vi "_Yt10_GoTo.vi"(11 "YTESTER测试数据":T1) -> (3 "YTESTER结论":T2)   [LabVIEW 2017]
doc: "VIClassID=YT_SSTEPFLAG_GOTO\nVIDescription=如果前面失败的话可以跳转某一位置进行重测，测试表也会更新掉。注意，也可以往后跳"
uses:
  YtCommon.lvlibp/yt`Step StepBaseInput.ctl
  YtCommon.lvlibp/yt`Step StepResult.ctl
  YtCommon.lvlibp/yt`Step TestData.ctl
  YtCommon.lvlibp/yt`Step System Queue.ctl
  YtCommon.lvlibp
panel:
  in  "YTESTER开放参数":T4={"YTESTER_BaseInput"={"isTest"=FALSE, "isSkip"=FALSE, "StepName"="Goto跳转器", "OnPass"=enum."Next", "OnFail"=enum."Next", "ReTestNumber"=0.0}, "跳转目标行(from1)"=1}
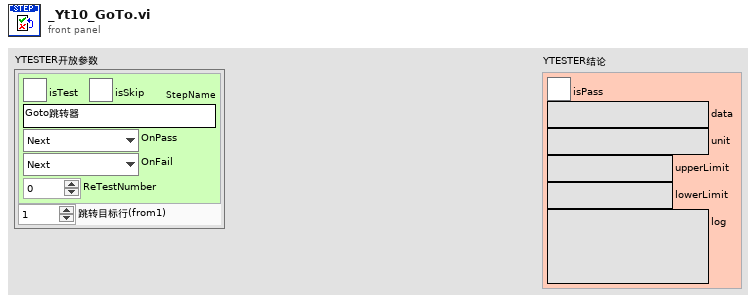
[diagram p1: front panel]
types:
  T1 = typedef "YtCommon.lvlibp/yt`Step TestData.ctl" = cluster{"Socket(From1)":i32, "SN":refnum<notifier>, "StopFlagRef":refnum<notifier>, "YT System Queue":refnum<queue>}
  T2 = typedef "YtCommon.lvlibp/yt`Step StepResult.ctl" = cluster{"isPass":bool, "data":string, "unit":string, "upperLimit":string, "lowerLimit":string, "log":string}
  T3 = typedef "YtCommon.lvlibp/yt`Step StepBaseInput.ctl" = cluster{"isTest":bool, "isSkip":bool, "StepName":string, "OnPass":enum16{"Next", "ToOVER", "Terminate"}, "OnFail":enum16{"Next", "ToOVER", "Terminate"}, "ReTestNumber":dbl}
  T4 = cluster{"YTESTER_BaseInput":T3, "跳转目标行(from1)":u32}
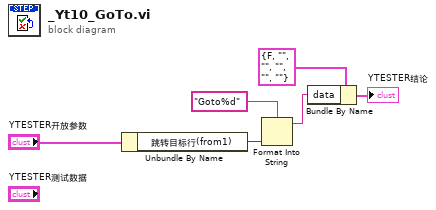
[diagram p0: block diagram]
diagram:
  n1 = Unbundle By Name("YTESTER开放参数") -> ("跳转目标行(from1)"=w3:u32)
  n2 = Format Into String(format string="Goto%d", w3) -> (resulting string=w1:string)  [unwired: 2 in, 1 out]
  n3 = Bundle By Name(cluster=T2 {"isPass"=FALSE, "data"="", "unit"="", "upperLimit"="", "lowerLimit"="", "log"=""} ("Result"), "data"=w1) -> (→"YTESTER结论":T2)
